vi "Ramsete Controller Simulation.vi"() -> ()   [LabVIEW 2019]
uses:
  Geometry/Typedef/Pose2d.ctl
  Geometry/Typedef/Translation2d.ctl
  Geometry/Typedef/Rotation2d.ctl
  Trajectory/Typedef/Differential Drive Constraints.ctl
  Trajectory/Typedef/Differential Drive Constants.ctl
  Trajectory/Typedef/Trajectory State.ctl
  <vilib>/Analysis/coordinate.llb/2D Cartesian Coordinate Rotation.vi
  <vilib>/Analysis/coordinate.llb/2D Cartesian Coordinate Rotation (Scalar).vi
panel:
  in  "index":i32
  out "states":T1[](array[typedef])
  out "Waveform Chart 6":dbl(graph)
  out "Waveform Chart 5":dbl(graph)
  out "Waveform Chart 4":dbl(graph)
  out "Waveform Chart 3":dbl(graph)
  out "Waveform Chart 2":dbl(graph)
  in  "Veloicty PID":T5={"kS"=0.2, "kV"=0.18, "kA"=0.1, "PIDF gains"={"Kp"=0.5, "Ki"=0.0, "Kd"=0.0, "Kf"=0.0}}
  out "Waveform Chart":T6(graph)
  out "Telemetry":cluster{dbl[], dbl[]}[](graph)
  in  "Config":T7={"Gear Reduction"=15.0, "Wheel Radius (m)"=0.076, "# Motors"=1, "coeff of friction"=0.1, "Mass (kg)"=50.0, "Motor"={"Ke (V)"=0.0183, "R (ohms)"=0.09, "KT (Nm/A)"=0.0183, "Tf (Nm)"=0.4}}
  in  "Turing Parameters":cluster{"b":dbl, "zeta":dbl}={"b"=2.0, "zeta"=0.7}
  out "Total Time Seconds":dbl
  in  "Constants":T8={"ks"=0.2, "kv"=0.18, "ka"=0.1, "trackwidth"=1.0}
  in  "Constraints":T9={"maxVoltage"=10.0, "maxVelocity"=5.0, "maxAccel"=10.0}
  in  "Waypoints":T2[](array[typedef])=[{"Translation2d"={"x"=0.0, "y"=0.0}, "Rotation2d"={"Theta"=0.0}}, {"Translation2d"={"x"=10.0, "y"=10.0}, "Rotation2d"={"Theta"=1.0}}, {"Translation2d"={"x"=30.0, "y"=40.0}, "Rotation2d"={"Theta"=0.5}}]
  out "Position":cluster{"X Out":dbl[], "Y Out":dbl[]}[](graph)
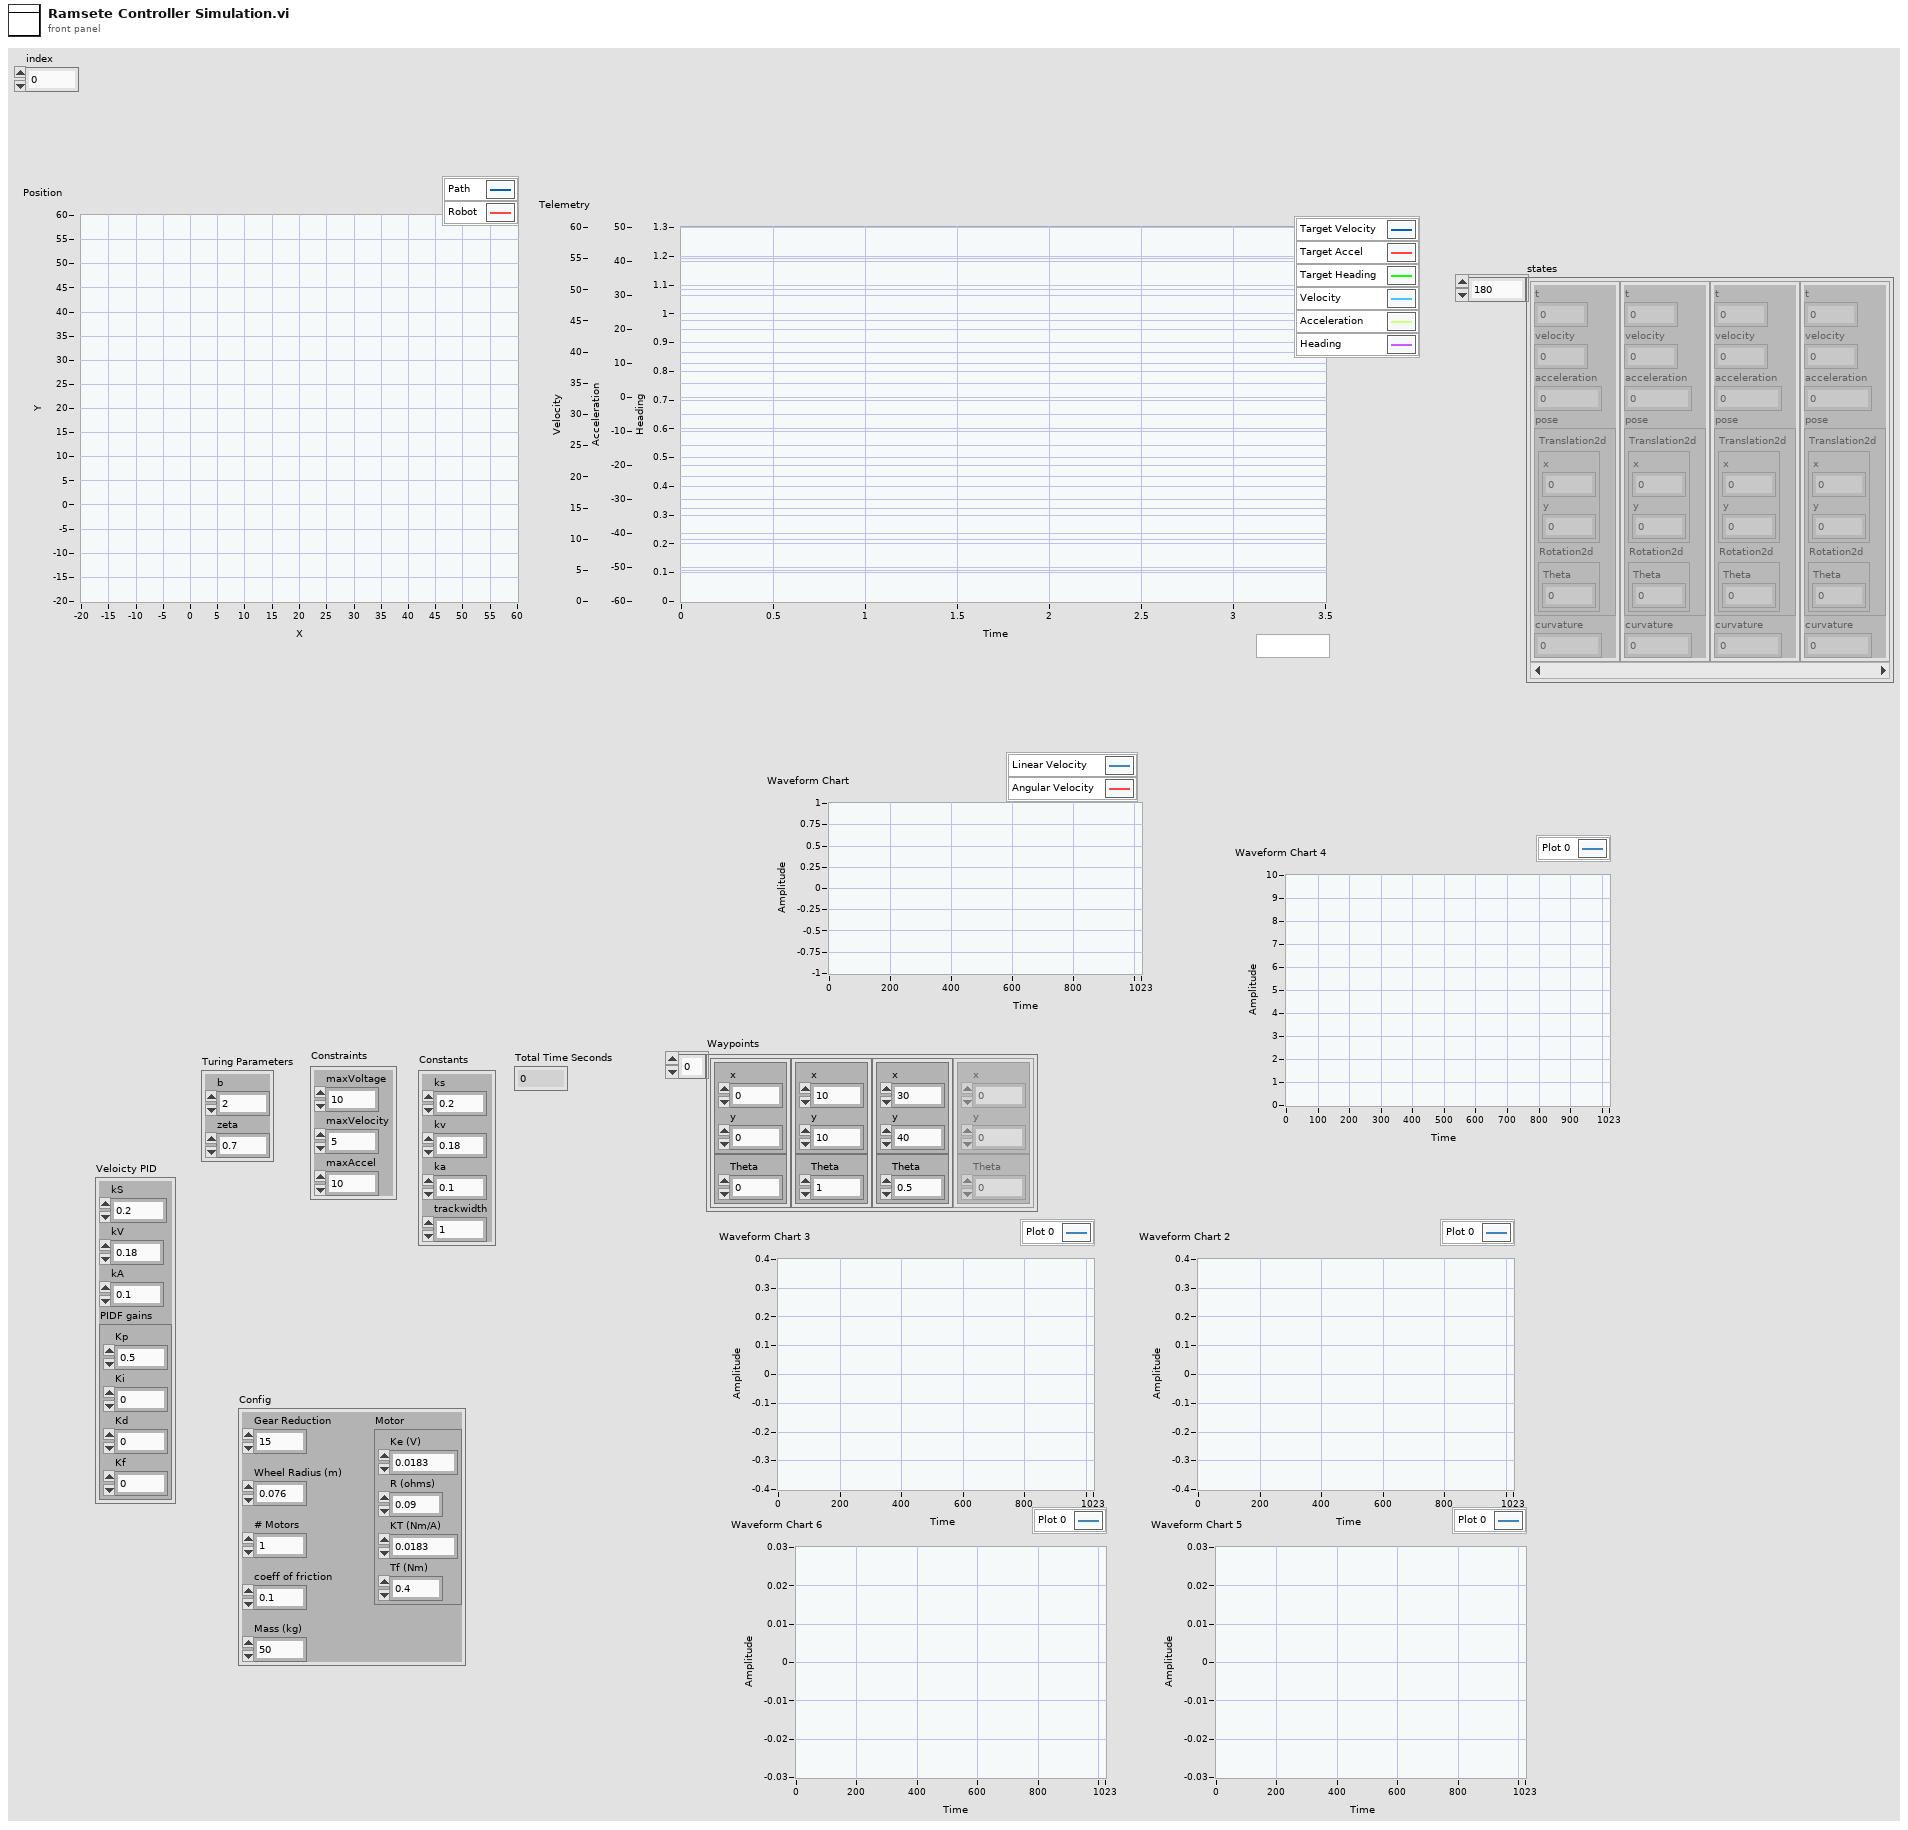
[diagram p1: front panel]
types:
  T1 = typedef "Trajectory State.ctl" = cluster{"t":dbl, "velocity":dbl, "acceleration":dbl, "pose":T2, "curvature":dbl}
  T2 = typedef "Pose2d.ctl" = cluster{"Translation2d":T3, "Rotation2d":T4}
  T3 = typedef "Translation2d.ctl" = cluster{"x":dbl, "y":dbl}
  T4 = typedef "Rotation2d.ctl" = cluster{"Theta":dbl}
  T5 = cluster{"kS":dbl, "kV":dbl, "kA":dbl, "PIDF gains":cluster{"Kp":dbl, "Ki":dbl, "Kd":dbl, "Kf":dbl}}
  T6 = cluster{"Linear Velocity":dbl, "Angular Velocity":dbl}
  T7 = cluster{"Gear Reduction":dbl, "Wheel Radius (m)":dbl, "# Motors":u32, "coeff of friction":dbl, "Mass (kg)":dbl, "Motor":cluster{"Ke (V)":dbl, "R (ohms)":dbl, "KT (Nm/A)":dbl, "Tf (Nm)":dbl}}
  T8 = typedef "Differential Drive Constants.ctl" = cluster{"ks":dbl, "kv":dbl, "ka":dbl, "trackwidth":dbl}
  T9 = typedef "Differential Drive Constraints.ctl" = cluster{"maxVoltage":dbl, "maxVelocity":dbl, "maxAccel":dbl}
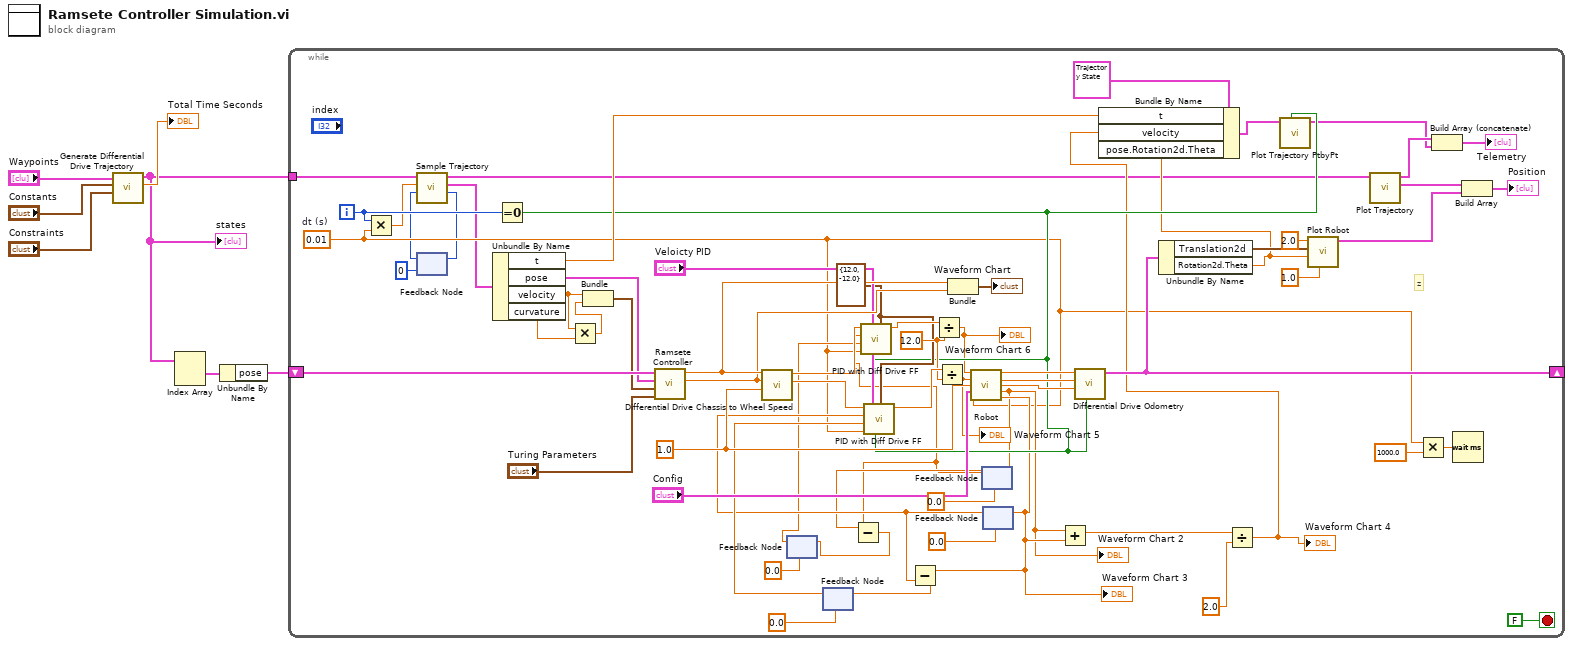
[diagram p0: block diagram]
diagram:
  n1 = call "Generate Differential Drive Trajectory.vi"("Constraints"="Constraints", "Constants"="Constants", "Waypoints"="Waypoints") -> ("Total Time Seconds"=→"Total Time Seconds":dbl, "states"=w1:T1[])  [unwired: 6 in, 1 out]
  "states" <- w1
  n2 = Index Array(array=w1) -> (element #1=w3:T1)  [unwired: 2 in, 1 out]
  n3 = Unbundle By Name(w3) -> ("pose"=w2:T2)
  n4 = while {
    shift-right: [w61] -> _
    shift-left: w2 -> [w70]
    tunnel: w1 -> [w15]
    i -> [w17]
    stop <- FALSE stop-if-true
    w16 = 0.01  # dt (s)
    w43 = cluster{"output high":dbl, "output low":dbl} {"output high"=12.0, "output low"=-12.0} ("output range")
    w44 = 12.0 ("x")
    w57 = 1.0 ("trackWidth")
    # "z"
    n5 = Multiply(x=w17, y=w16) -> (x*y=w12:dbl)
    n6 = feedback #1(0 ("index")) -> (w8:i32)
    n7 = call "Sample Trajectory.vi"("start index (0)"=w8, "timestamp"=w12, "Trajectory States"=w15) -> ("index"=w11:i32, "State"=w13:T1, "Trajectory States out"=w14:T1[])  [unwired: 6 in]
    n8 = feedback-in #1(w11) -> ()
    n9 = Unbundle By Name(w13) -> ("t"=w38:dbl, "pose"=w69:T2, "velocity"=w29:dbl, "curvature"=w30:dbl)
    n10 = Equal To 0?(x=w17) -> (x = 0?=w36:bool)
    n11 = Multiply(x=w29, y=w30) -> (x*y=w28:dbl)
    n12 = Bundle("velocity"=w29, w28) -> (w67:cluster{"velocity":dbl, dbl})  [unwired: 1 in]
    n13 = call "Ramsete Controller.vi"("Turing Parameters"="Turing Parameters", "Velocity Ref"=w67, "Pose Ref"=w69, "Current Pose"=w70) -> ("Angular Velocity"=w56:dbl, "Linear Velocity"=w59:dbl)  [unwired: 6 in]
    n14 = call "Differential Drive Chassis to Wheel Speed.vi"("trackWidth"=w57, "omega"=w56, "vx"=w59) -> ("right"=w52:dbl, "left"=w53:dbl)  [unwired: 7 in]
    n15 = feedback #2(0.0 ("Right Velocity")) -> (w18:dbl)
    n16 = feedback #3(0.0 ("Right Velocity")) -> (w25:dbl)
    n17 = Bundle("Linear Velocity"=w59, "Angular Velocity"=w56) -> (→"Waveform Chart":T6)  [unwired: 1 in]
    n18 = feedback #4(0.0 ("Right Velocity")) -> (w20:dbl)
    n19 = call "PID with Diff Drive FF.vi"("output range"=w43, "reinitialize? (F)"=w36, "Feed Forward Constants"="Veloicty PID", "dt (s)"=w16, "Acceleration (0)"=w18, "Velocity"=w20, "Velocity Reference"=w53) -> ("Output"=w50:dbl)  [unwired: 4 in]
    n20 = Divide(x=w50, y=w44) -> (x/y=w32:dbl)
    "Waveform Chart 6" <- w32
    n21 = feedback #5(0.0 ("Right Velocity")) -> (w23:dbl)
    n22 = call "PID with Diff Drive FF.vi"("output range"=w43, "reinitialize? (F)"=w36, "Feed Forward Constants"="Veloicty PID", "dt (s)"=w16, "Acceleration (0)"=w25, "Velocity"=w23, "Velocity Reference"=w52) -> ("Output"=w49:dbl)  [unwired: 4 in]
    n23 = Divide(x=w49, y=w44) -> (x/y=w31:dbl)
    "Waveform Chart 5" <- w31
    n24 = call "Robot.vi"("Left Value"=w32, "Right Value"=w31, "WheelBase"=w57, "Config"="Config", "dt (s)"=w16) -> ("Left Distance"=w48:dbl, "Right Distance"=w47:dbl, "Angle"=w71:dbl, "Left Velocity"=w21:dbl, "Right Velocity"=w24:dbl)  [unwired: 6 in]
    "Waveform Chart 2" <- w21
    "Waveform Chart 3" <- w24
    n25 = Subtract(x=w21, y=w20) -> (x-y=w19:dbl)
    n26 = feedback-in #2(w19) -> ()
    n27 = Subtract(x=w24, y=w23) -> (x-y=w22:dbl)
    n28 = feedback-in #3(w22) -> ()
    n29 = feedback-in #4(w21) -> ()
    n30 = feedback-in #5(w24) -> ()
    n31 = Add(x=w21, y=w24) -> (x+y=w42:dbl)
    n32 = call "Differential Drive Odometry.vi"("Reset"=w36, "Theta"=w71, "Right Distance"=w47, "Left Distance"=w48) -> ("Pose"=w61:T2)  [unwired: 7 in]
    n33 = Unbundle By Name(w61) -> ("Translation2d"=w73:T3, "Rotation2d.Theta"=w33:dbl)
    n34 = Divide(x=w42, y=2.0) -> (x/y=w34:dbl)
    "Waveform Chart 4" <- w34
    n35 = Bundle By Name(cluster=T1 {"t"=0.0, "velocity"=0.0, "acceleration"=0.0, "pose"={"Translation2d"={"x"=0.0, "y"=0.0}, "Rotation2d"={"Theta"=0.0}}, "curvature"=0.0} ("State"), "t"=w38, "velocity"=w34, "pose.Rotation2d.Theta"=w33) -> (w37:T1)
    n36 = call "Plot Trajectory PtbyPt.vi"("Reset? (F)"=w36, "State"=w37) -> ("Telemetry"=w35:cluster{dbl[], dbl[]}[])  [unwired: 9 in]
    n37 = call "Plot Robot.vi"("Length"=1.0, "Angle"=w33, "Location"=w73, "Width"=2.0) -> ("Cluster"=w64:cluster{"X Out":dbl[], "Y Out":dbl[]})  [unwired: 7 in]
    n38 = call "Plot Trajectory.vi"("states"=w14) -> ("Position"=w65:cluster{dbl[], dbl[]}, "Telemetry"=w62:cluster{dbl[], dbl[]}[])  [unwired: 9 in]
    n39 = Multiply(x=w16, y=1000.0) -> (x*y=w55:dbl)
    n40 = Build Array (concatenate)(w62, w35) -> (→"Telemetry":cluster{dbl[], dbl[]}[])
    n41 = Wait (ms)(milliseconds to wait=w55) -> ()  [unwired: 1 out]
    n42 = Build Array(w65, w64) -> (→"Position":cluster{"X Out":dbl[], "Y Out":dbl[]}[])
  }
